vi "Table Read.vi"(4 "error in (no error)":errorcluster, 5 "Type of Anything":variant, 6 "Container State":T4, 7 "Display State In":T1) -> (0 "error out":errorcluster, 2 "Value":variant, 3 "Display State Out":T1)   [LabVIEW 2015, in "KTable.xctl"]
uses:
  KTable.xctl
  <vilib>/_xctls/Container State.ctl
  State.ctl
  ColumnSpec.ctl
  ColumnType.ctl
  <vilib>/_xctls/XControlSupport.lvlib
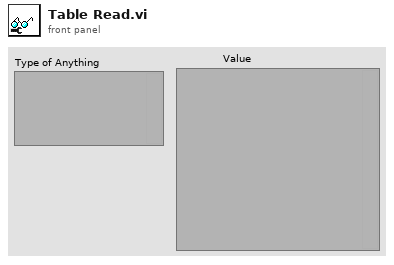
[diagram p1: front panel]
types:
  T1 = typedef "KTable.xctl/State.ctl" = cluster{"Columns":T2[], "Listbox":refnum<vi>}
  T2 = typedef "KTable.xctl/ColumnSpec.ctl" = cluster{"Name":string, "Type":T3, "Width":i32, "Strings":string[]}
  T3 = typedef "KTable.xctl/ColumnType.ctl" = enum16{"String", "Enum", "Int", "Double", "Boolean", "Ring"}
  T4 = typedef "XControlSupport.lvlib/Container State.ctl" = cluster{"Indicator?":bool, "Run Mode?":bool, " Refnum":refnum<vi>}
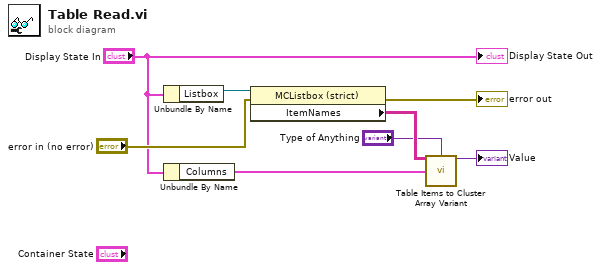
[diagram p0: block diagram]
diagram:
  n1 = Unbundle By Name("Display State In") -> ("Listbox"=w8:refnum<vi>)
  n2 = Unbundle By Name("Display State In") -> ("Columns"=w3:T2[])
  n3 = property class="MCListbox (strict)"(reference=w8, error in="error in (no error)") -> (error out=→"error out":errorcluster, "ItemNames"=w4:string[][])  [unwired: 1 out]
  n4 = call "Table Items to Cluster Array Variant.vi"("Table Items"=w4, "Type of Anything"="Type of Anything", "Columns"=w3) -> ("Anything"=→"Value":variant)  [unwired: 11 in, 1 out]
  "Display State Out" <- "Display State In"
